vi "Global - Client.vi"() -> ()   [LabVIEW 2024]
doc: "Stores the global data for the client."
panel:
  in  "Logging Database URL":path=path "\\\\localhost\\c__archive"
  in  "Archive Database URL":path=path "\\\\localhost\\c__data"
  # "The Global - Client.vi stores the global data for the client. The global data includes the static configurations and data that are not changed frequently and can be visited from anywhere in the code."
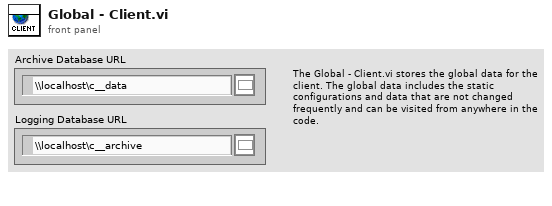
[diagram p1: front panel]
diagram:
